vi "Write_raw_data.vi"(4 "error in":errorcluster, 5 "image_data":u16[][][](array[numeric]), 6 "sequencer":T1(array[cluster]), 7 "ref in":i32) -> (0 "error out":errorcluster, 3 "ref out":i32)   [LabVIEW 2010]
uses:
  <vilib>/addons/h5labview2/base/hid_t.ctl
  <vilib>/addons/h5labview2/dataset/H5Dwrite.llb/H5Dwrite.xnode
  <vilib>/addons/h5labview2/attrib/H5Awrite.llb/H5Awrite.xnode
  <vilib>/addons/h5labview2/base/lib_path.vi
  <vilib>/addons/h5labview2/base/H5Equery.vi
  <vilib>/addons/h5labview2/group/H5G.lvlib
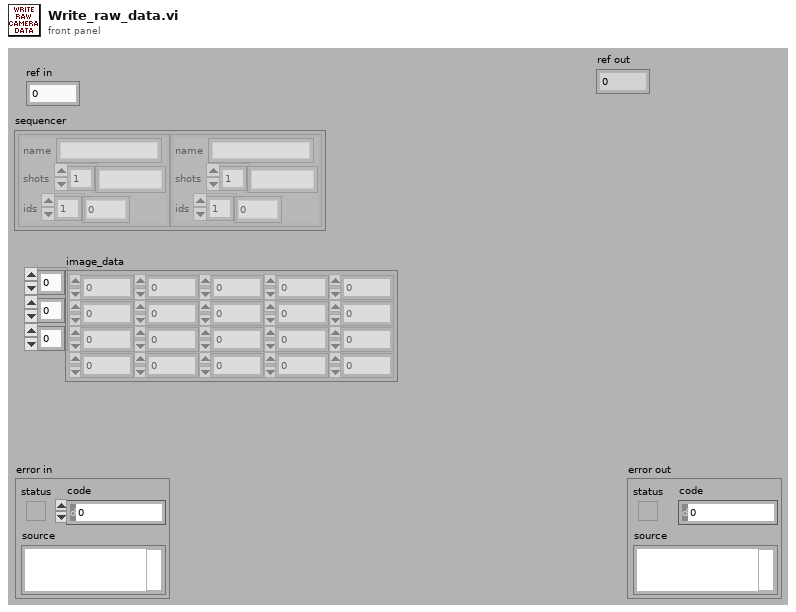
[diagram p1: front panel]
types:
  T1 = cluster{"name":string, "shots":string[], "ids":i32[]}[]
  T2 = typedef "hid_t.ctl" = i32
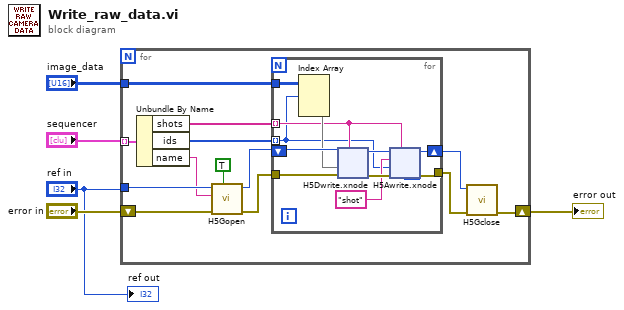
[diagram p0: block diagram]
diagram:
  n1 = for {
    tunnel: "image_data" -> [w18]
    tunnel: "sequencer" -> [w17] mode=indexing
    shift-right: [w7] -> w2
    shift-left: "error in" -> [w11]
    tunnel: "ref in" -> [w14]
    n2 = Unbundle By Name(w17) -> ("shots"=w16:string[], "ids"=w15:i32[], "name"=w13:string)
    n3 = call <vilib>:"H5Gopen.vi"("create? (F)"=TRUE ("Create if not found (F)"), "error in (no error)"=w11, "name"=w13, "ref in"=w14) -> ("error out"=w10:errorcluster, "group out"=w9:T2)  [unwired: 6 in]
    n4 = for {
      tunnel: w10 -> [w27]
      tunnel: w18 -> [w29]
      tunnel: w16 -> [w22] mode=indexing
      tunnel: w15 -> [w21] mode=indexing
      tunnel: [w20] -> w8
      shift-right: [w19] -> w6
      shift-left: w9 -> [w28]
      n5 = Index Array(array=w29, index (dim 0)=w21) -> (element=w24:u16[][])  [unwired: 2 in]
      n6 = xnode "H5Dwrite.xnode"("dataset name"=w22, "error in (no error)"=w27, "data"=w24, "ref in"=w28) -> ("error out"=w26:errorcluster, "ref out"=w25:T2)  [unwired: 3 in, 1 out]
      n7 = xnode "H5Awrite.xnode"("object name"=w22, "error in (no error)"=w26, "data"=w21, "attrib name"="shot" ("attribute"), "ref in"=w25) -> ("error out"=w20:errorcluster, "ref out"=w19:T2)  [unwired: 2 in, 1 out]
    }
    n8 = call <vilib>:"H5Gclose.vi"("error in (no error)"=w8, "group in"=w6) -> ("error out"=w7:errorcluster)  [unwired: 9 in]
  }
  "error out" <- w2
  "ref out" <- "ref in"
